vi "Check_Box_valid.vi"(1 "Box to check":T1=[{"Max"=16000.0, "Min"=14000.0}, {"Max"=1000.0, "Min"=-1000.0}, {"Max"=700.0, "Min"=0.0}] {"Min" format="%#.1f"; "Max" format="%#.1f"}) -> (0 "Valid Box":bool)   [LabVIEW 2010]
uses:
  Box_size.ctl
panel:
  # "X                           Y                          Z"
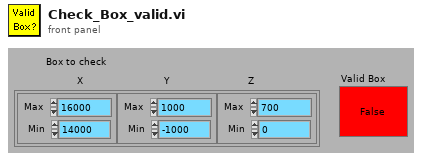
[diagram p1: front panel]
types:
  T1 = typedef "Box_size.ctl" = cluster{"Max":dbl, "Min":dbl}[]
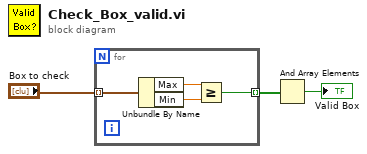
[diagram p0: block diagram]
diagram:
  n1 = for {
    tunnel: "Box to check" -> [w7] mode=indexing
    tunnel: [w4] -> w1 mode=indexing
    n2 = Unbundle By Name(w7) -> ("Max"=w6:dbl, "Min"=w5:dbl)
    n3 = Greater Or Equal?(x=w6, y=w5) -> (x >= y?=w4:bool)
  }
  n4 = And Array Elements(Boolean array=w1) -> (logical AND=→"Valid Box":bool)
